vi "Load Settings from XML.vi"(8 "error in (no error)":errorcluster, 11 "Settings in":T1) -> (0 "error out":errorcluster, 3 "Settings out":T1)   [LabVIEW 2017, in "Settings.lvlib"]
doc: "Attempts to load previous user specified settings from an XML file.\n\nThis VI will not generate an error. If a suitable XML file can't be loaded and parsed then it will simply return the default settings."
uses:
  Settings.lvlib
  Settings.ctl
  Acquisition/Hardware Configuration.ctl
  <vilib>/Utility/xml.llb/Read From XML File(string).vi
  <vilib>/Utility/xml.llb/Write to XML File(string).vi
  Acquisition/Acquisition.lvlib
panel:
  # "(Scroll up for Settings Controls)"
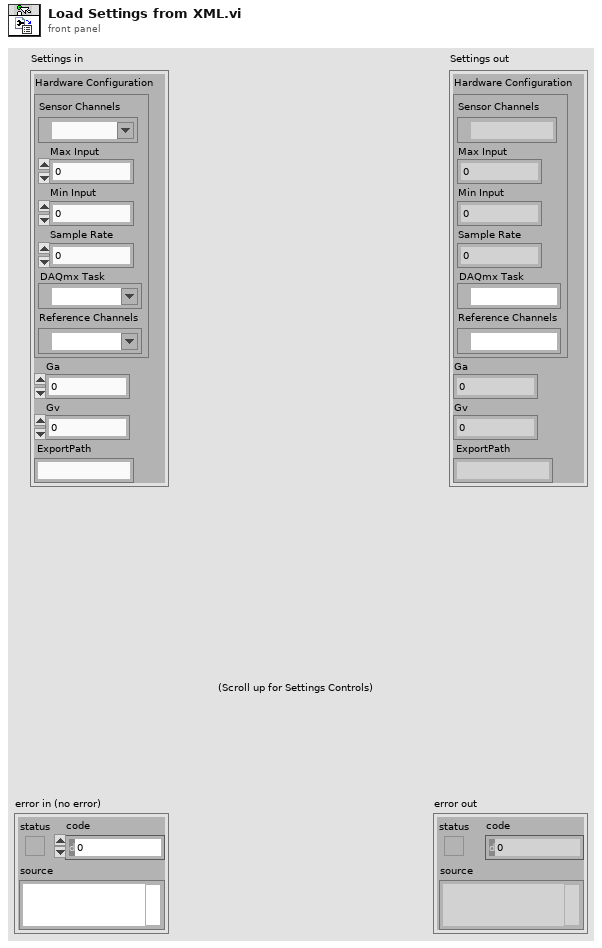
[diagram p1: front panel]
types:
  T1 = typedef "Settings.lvlib/Settings.ctl" = cluster{"Hardware Configuration":T2, "Ga":dbl, "Gv":dbl, "ExportPath":string}
  T2 = typedef "Acquisition.lvlib/Hardware Configuration.ctl" = cluster{"Sensor Channels":tag, "Max Input":dbl, "Min Input":dbl, "Sample Rate":dbl, "DAQmx Task":refnum<k21>, "Reference Channels":tag}
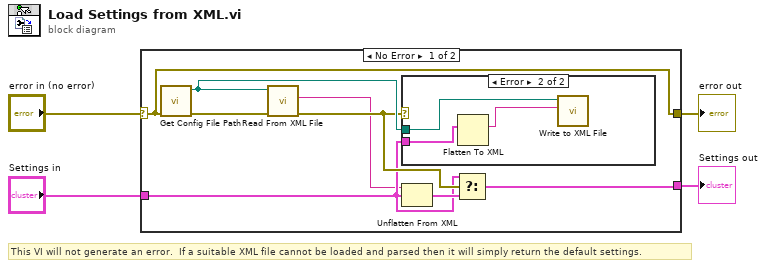
[diagram p0: block diagram]
diagram:
  # "This VI will not generate an error.  If a suitable XML file cannot be loaded and parsed then it will simply return the default settings."
  n1 = case shown="No Error" "error in (no error)" {
    selector: "error in (no error)" -> [w12 w17]
    tunnel: [w12 w17] -> w3
    tunnel: "Settings in" -> [w7 w16]
    tunnel: [w5 w16] -> w1
    frame No Error {
      n2 = call "Get Config File Path.vi"("error in (no error)"=w12) -> ("error out"=w11:errorcluster, "XML File Path"=w10:path)  [unwired: 9 in]
      n3 = call-poly <vilib>:"Read From XML File.vi"("error in (no error)"=w11, "XML File Path"=w10) -> ("error out"=w9:errorcluster, "XML Elements"=w6:string)  [unwired: 7 in, 1 out]
      n4 = case shown="Error" w9 {
        tunnel: w7 -> [_ w15]
        tunnel: w10 -> [_ w13]
        frame No Error {
        }
        frame Error {
          n5 = Flatten To XML(anything=w15) -> (xml string=w14:string)
          n6 = call-poly <vilib>:"Write to XML File.vi"("XML Input"=w14, "XML File Path"=w13) -> ()  [unwired: 7 in, 3 out]
        }
      }
      n7 = Unflatten From XML(xml string=w6, type=w7) -> (value=w8:T1)  [unwired: 1 in, 1 out]
      n8 = Select(t=w7, s=w9, f=w8) -> (s? t:f=w5:T1)
    }
    frame Error {
    }
  }
  "error out" <- w3
  "Settings out" <- w1
